vi "Query Resource Access Information - 1Pin MRsrc.vi"(7 "sites":i32[](array[numeric]), 8 "error in (no error)":errorcluster, 9 "instrument type id":string, 10 "pin or relay name":string, 11 "pin map id":string) -> (0 "error out":errorcluster, 2 "resource access information":T1[](array[typedef]))   [LabVIEW 2020, in "MeasurementLink Pin Map.lvlib"]
doc: "Queries the pin map service for resouce access information for the specified <b>pin or relay name</b>, <b>instrument type</b>, and <b>sites</b>. This information can be used to map a single pin across multiple sites to the associated hardware resources and connections used to make measurements on that pin."
uses:
  MeasurementLink Pin Map.lvlib
  MeasurementLink Pin Map Client/RPC Messages/ni_measurementlink_pinmap_v1_ResourceAccessInformation.ctl
  MeasurementLink Pin Map Client/RPC Messages/ni_measurementlink_pinmap_v1_ChannelMapping.ctl
  MeasurementLink Pin Map Client/MeasurementLink Pin Map Client.lvlib
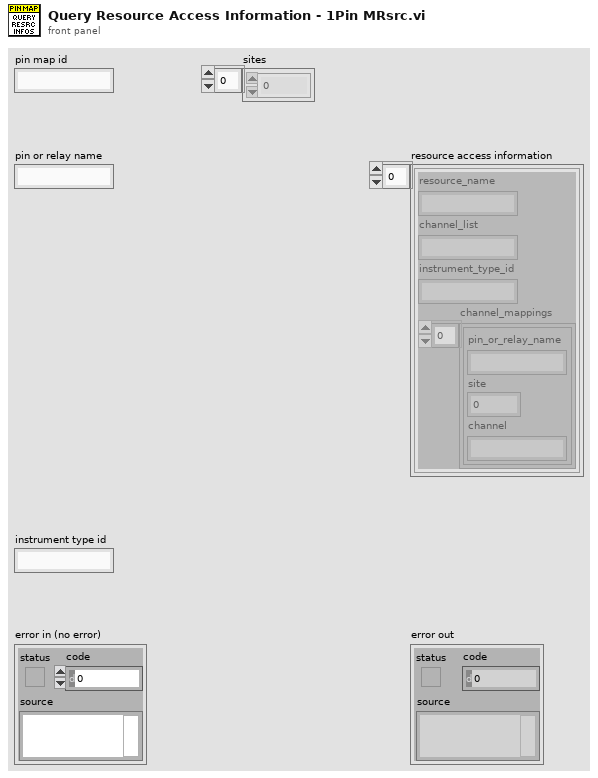
[diagram p1: front panel]
types:
  T1 = typedef "MeasurementLink Pin Map Client.lvlib/ni_measurementlink_pinmap_v1_ResourceAccessInformation.ctl" = cluster{"resource_name":string, "channel_list":string, "instrument_type_id":string, "channel_mappings":T2[]}
  T2 = typedef "MeasurementLink Pin Map Client.lvlib/ni_measurementlink_pinmap_v1_ChannelMapping.ctl" = cluster{"pin_or_relay_name":string, "site":i32, "channel":string}
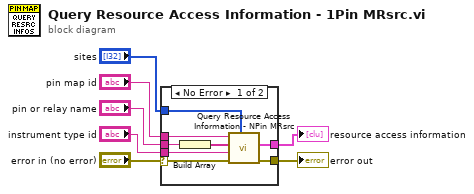
[diagram p0: block diagram]
diagram:
  n1 = case shown="No Error" "error in (no error)" {
    selector: "error in (no error)" -> [w15 w16]
    tunnel: "pin or relay name" -> [w13 _]
    tunnel: "instrument type id" -> [w10 _]
    tunnel: [w14 w16] -> w5
    tunnel: [w11 _] -> w3
    tunnel: "pin map id" -> [w9 _]
    tunnel: "sites" -> [w8 _]
    frame No Error {
      n2 = Build Array(w13) -> (w12:string[])
      n3 = call "Query Resource Access Information - NPin MRsrc.vi"("sites"=w8, "error in (no error)"=w15, "instrument type id"=w10, "pin or relay names"=w12, "pin map id"=w9) -> ("error out"=w14:errorcluster, "resource access information"=w11:T1[])  [unwired: 5 in]
    }
    frame Error {
    }
  }
  "error out" <- w5
  "resource access information" <- w3
